vi "Replace Project PPLs.vi"(8 "error in":errorcluster, 9 "CD lvproj name":string, 10 "CD name":string, 11 "custom device path":path) -> (0 "error out":errorcluster, 3 "custom device path out":path)   [LabVIEW 2020, in "Template Tool.lvlib"]
uses:
  Template Tool.lvlib
panel:
  out "VIs relinked":string[](array[string])
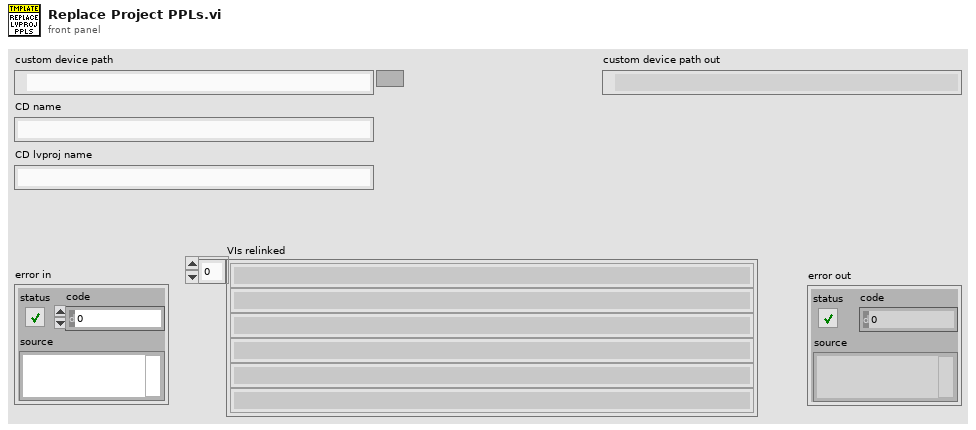
[diagram p1: front panel]
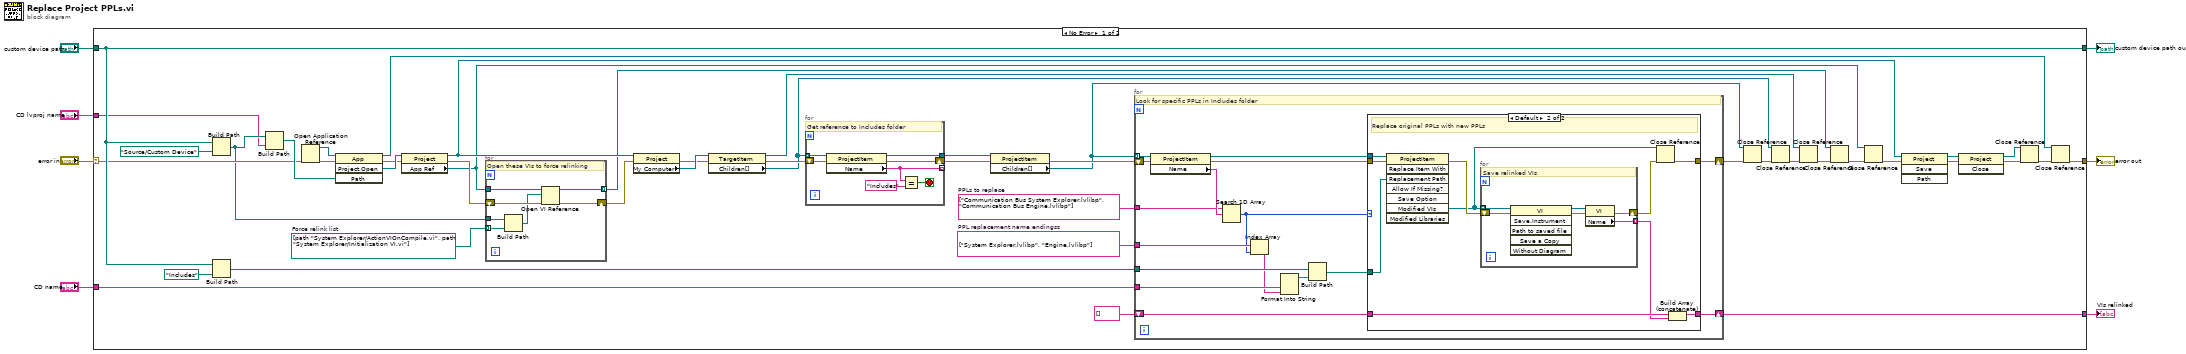
[diagram p0: block diagram]
diagram:
  n1 = case shown="No Error" "error in" {
    selector: "error in" -> [w32 w102]
    tunnel: "custom device path" -> [w33 w101]
    tunnel: [w36 _] -> w6
    tunnel: [w18 w102] -> w5
    tunnel: [w33 w101] -> w4
    tunnel: "CD lvproj name" -> [w9 _]
    tunnel: "CD name" -> [w8 _]
    frame No Error {
      w23 = path[] [path "System Explorer/ActionVIOnCompile.vi", path "System Explorer/Initialization VI.vi"]  # Force relink list
      w38 = string[] ["System Explorer.lvlibp", "Engine.lvlibp"]  # PPL replacement name endingss
      w39 = string[] ["Communication Bus System Explorer.lvlibp", "Communication Bus Engine.lvlibp"]  # PPLs to replace
      n2 = Build Path(base path=w33, name or relative path=path "Source/Custom Device") -> (appended path=w24:path)
      n3 = Build Path(base path=w33, name or relative path=path "Includes") -> (appended path=w15:path)
      n4 = Build Path(base path=w24, name or relative path=w9) -> (appended path=w47:path)
      n5 = Open Application Reference(8:w32) -> (0:w14:errorcluster, 3:w51:refnum<vi>)  [unwired: 3 in]
      n6 = invoke class="App" method="Project.Open"(reference=w51, error in=w14, "Path"=w47) -> (reference out=w17:refnum<vi>, error out=w30:errorcluster, "Project:Open"=w31:refnum<vi>)  [unwired: 1 in, 1 out]
      n7 = property class="Project"(reference=w31, error in=w30) -> (reference out=w27:refnum<vi>, error out=w29:errorcluster, "App Ref"=w20:refnum<vi>)
      n8 = for {
        tunnel: w20 -> [w59]
        tunnel: [w54] -> w25 mode=indexing
        tunnel: w24 -> [w57]
        tunnel: w23 -> [w56] mode=indexing
        shift-right: [w53] -> w28
        shift-left: w29 -> [w58]
        # "Open these VIs to force relinking"
        n9 = Build Path(base path=w57, name or relative path=w56) -> (appended path=w55:path)
        n10 = Open VI Reference(application reference (local)=w59, vi path=w55, error in (no error)=w58) -> (vi reference=w54:refnum<vi>, error out=w53:errorcluster)  [unwired: 3 in]
      }
      n11 = property class="Project"(reference=w27, error in=w28) -> (error out=w44:errorcluster, "My Computer"=w45:refnum<vi>)  [unwired: 1 out]
      n12 = property class="TargetItem"(reference=w45, error in=w44) -> (reference out=w43:refnum<vi>, error out=w50:errorcluster, "Children[]"=w34:refnum<vi>[])
      n13 = for {
        tunnel: w34 -> [w100] mode=indexing
        tunnel: [w99] -> _ mode=indexing
        tunnel: [w96] -> w40
        shift-right: [w94] -> w46
        shift-left: w50 -> [w95]
        stop <- w97 stop-if-true
        # "Get reference to Includes folder"
        n14 = property class="ProjectItem"(reference=w100, error in=w95) -> (reference out=w96:refnum<vi>, error out=w94:errorcluster, "Name"=w99:string)
        n15 = Equal?(x=w99, y="Includes") -> (x = y?=w97:bool)
      }
      n16 = property class="ProjectItem"(reference=w40, error in=w46) -> (error out=w49:errorcluster, "Children[]"=w35:refnum<vi>[])  [unwired: 1 out]
      n17 = for {
        tunnel: w35 -> [w75] mode=indexing
        shift-right: [w66] -> w48
        shift-left: w49 -> [w74]
        tunnel: w39 -> [w72]
        tunnel: w38 -> [w69]
        shift-right: [w64] -> w36
        shift-left: string[] [] -> [w65]
        tunnel: w8 -> [w62]
        tunnel: w15 -> [w63]
        # "Look for specific PPLs in Includes folder"
        n18 = property class="ProjectItem"(reference=w75, error in=w74) -> (reference out=w71:refnum<vi>, error out=w70:errorcluster, "Name"=w73:string)
        n19 = Search 1D Array(1D array=w72, element=w73) -> (index of element=w68:i32)  [unwired: 1 in]
        n20 = Index Array(array=w69, index=w68) -> (element=w61:string)
        n21 = Format Into String(w62, w61) -> (resulting string=w60:string)  [unwired: 3 in, 1 out]
        n22 = Build Path(base path=w63, name or relative path=w60) -> (appended path=w67:path)
        n23 = case shown="Default" w68 {
          tunnel: w71 -> [_ w87]
          tunnel: w70 -> [w77 w86]
          tunnel: w67 -> [_ w85]
          tunnel: [w77 w82] -> w66
          tunnel: w65 -> [w76 w80]
          tunnel: [w76 w78] -> w64
          frame -1 {
          }
          frame Default {
            # "Replace original PPLs with new PPLs"
            n24 = invoke class="ProjectItem" method="Replace Item With"(reference=w87, error in=w86, "Replacement Path"=w85) -> (error out=w84:errorcluster, "Modified VIs"=w81:refnum<vi>[])  [unwired: 5 in, 6 out]
            n25 = for {
              tunnel: w81 -> [w91] mode=indexing
              shift-right: [w89] -> w83
              shift-left: w84 -> [w90]
              tunnel: [w88] -> w79 mode=indexing
              # "Save relinked VIs"
              n26 = invoke class="VI" method="Save.Instrument"(reference=w91, error in=w90) -> (reference out=w93:refnum<vi>, error out=w92:errorcluster)  [unwired: 4 in, 4 out]
              n27 = property class="VI"(reference=w93, error in=w92) -> (error out=w89:errorcluster, "Name"=w88:string)  [unwired: 1 out]
            }
            n28 = Close Reference(reference=w81, error in (no error)=w83) -> (error out=w82:errorcluster)
            n29 = Build Array (concatenate)(w80, w79) -> (w78:string[])
          }
        }
      }
      n30 = Close Reference(reference=w35, error in (no error)=w48) -> (error out=w41:errorcluster)
      n31 = Close Reference(reference=w34, error in (no error)=w41) -> (error out=w42:errorcluster)
      n32 = Close Reference(reference=w43, error in (no error)=w42) -> (error out=w26:errorcluster)
      n33 = Close Reference(reference=w25, error in (no error)=w26) -> (error out=w22:errorcluster)
      n34 = Close Reference(reference=w20, error in (no error)=w22) -> (error out=w21:errorcluster)
      n35 = invoke class="Project" method="Save"(reference=w27, error in=w21) -> (reference out=w12:refnum<vi>, error out=w11:errorcluster)  [unwired: 2 in, 2 out]
      n36 = invoke class="Project" method="Close"(reference=w12, error in=w11) -> (reference out=w13:refnum<vi>, error out=w10:errorcluster)  [unwired: 1 in, 1 out]
      n37 = Close Reference(reference=w13, error in (no error)=w10) -> (error out=w19:errorcluster)
      n38 = Close Reference(reference=w17, error in (no error)=w19) -> (error out=w18:errorcluster)
    }
    frame Error {
    }
  }
  "error out" <- w5
  "custom device path out" <- w4
  "VIs relinked" <- w6
